vi "GEA3 HEWH Example.vi"() -> ()   [LabVIEW 2016]
uses:
  type defs/ERD Write Data In.ctl
  type defs/Data Type.ctl
  Type Definitions/GEA3 HEWH ERD Data.ctl
  Type Definitions/GEA3 HEWH Mixing Valve.ctl
  library/GEA2_Toolkit.lvlib
panel:
  in  "index":i32
  in  "Enable EMV List":bool
  out "ERD Data":string[][](array[string])
  out "Cycles":i32
  out "ERD Data":T1
  out "Raw Data Out":string
  in  "ERD Write Data In":T3 {"ERD Number" format="%.0x"}
  in  "Configure Send?":bool
  in  "stop":bool
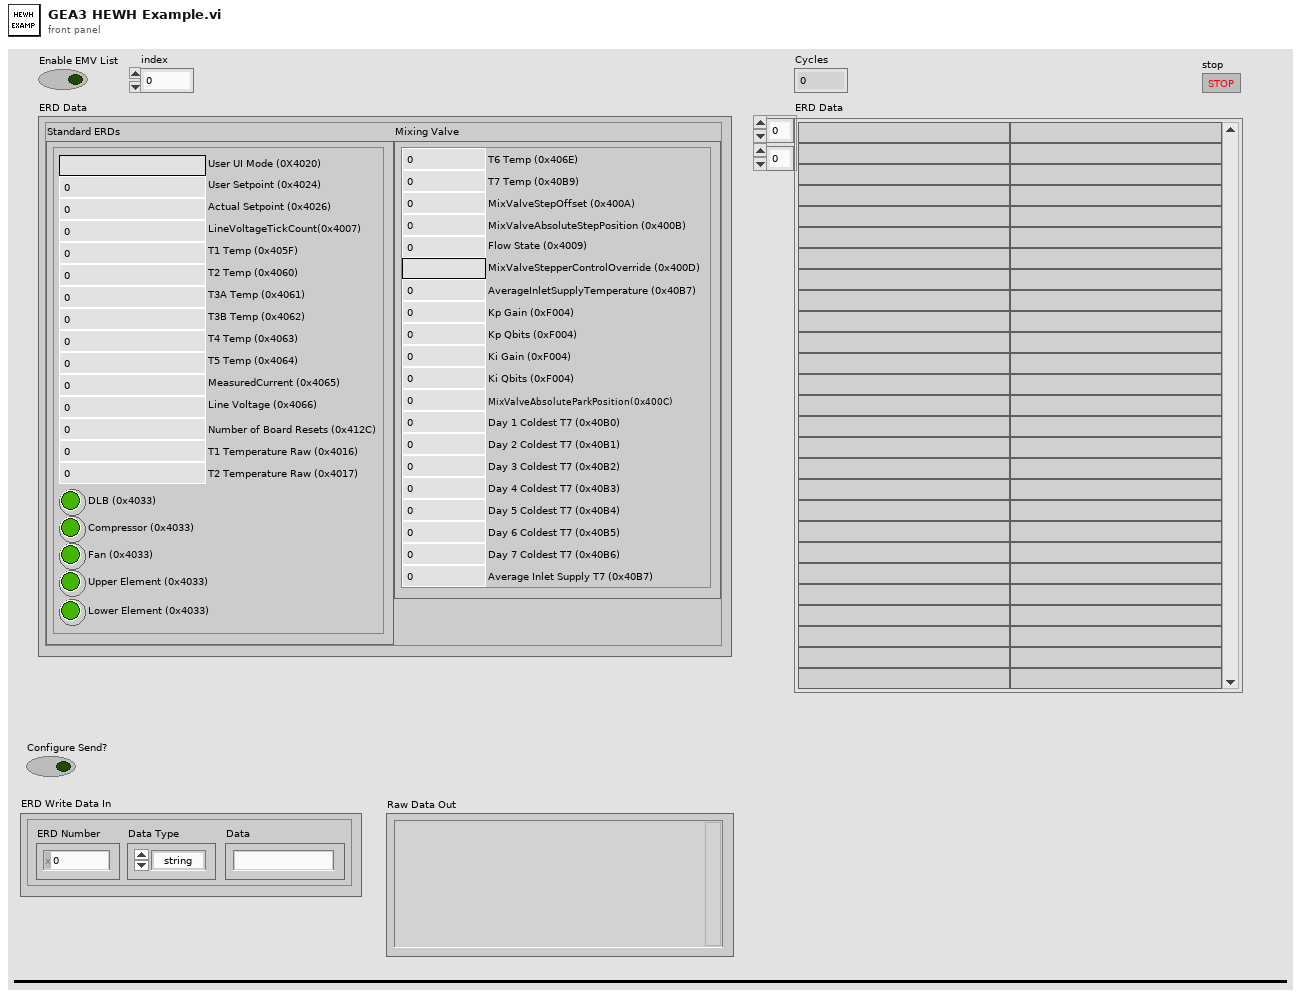
[diagram p1: front panel]
types:
  T1 = typedef "GEA3 HEWH ERD Data.ctl" = cluster{"Mixing Valve":T2, "Standard ERDs":cluster{"User UI Mode (0X4020)":string, "User Setpoint (0x4024)":u16, "Actual Setpoint (0x4026)":u16, "DLB (0x4033)":bool, "Compressor (0x4033)":bool, "Lower Element (0x4033)":bool, "Upper Element (0x4033)":bool, "Fan (0x4033)":bool, "T1 Temp (0x405F)":dbl, "T2 Temp (0x4060)":dbl, "T3A Temp (0x4061)":dbl, "T3B Temp (0x4062)":dbl, "T4 Temp (0x4063)":dbl, "T5 Temp (0x4064)":dbl, "Line Voltage (0x4066)":dbl, "MeasuredCurrent (0x4065)":dbl, "LineVoltageTickCount(0x4007)":u16, "Number of Board Resets (0x412C)":u16, "T1 Temperature Raw (0x4016)":u16, "T2 Temperature Raw (0x4017)":u16}}
  T2 = typedef "GEA3 HEWH Mixing Valve.ctl" = cluster{"T7 Temp (0x40B9)":dbl, "MixValveStepOffset (0x400A)":i16, "MixValveAbsoluteStepPosition (0x400B)":i16, "Flow State (0x4009)":u8, "MixValveStepperControlOverride (0x400D)":string, "AverageInletSupplyTemperature (0x40B7)":dbl, "T6 Temp (0x406E)":dbl, "Kp Gain (0xF004)":u16, "Kp Qbits (0xF004)":u16, "Ki Gain (0xF004)":u16, "Ki Qbits (0xF004)":u16, "MixValveAbsoluteParkPosition(0x400C)":i16, "Day 2 Coldest T7 (0x40B1)":dbl, "Day 1 Coldest T7 (0x40B0)":dbl, "Day 4 Coldest T7 (0x40B3)":dbl, "Day 3 Coldest T7 (0x40B2)":dbl, "Day 6 Coldest T7 (0x40B5)":dbl, "Day 5 Coldest T7 (0x40B4)":dbl, "Average Inlet Supply T7 (0x40B7)":dbl, "Day 7 Coldest T7 (0x40B6)":dbl}
  T3 = typedef "GEA2_Toolkit.lvlib/ERD Write Data In.ctl" = cluster{"ERD Number":u16, "Data Type":T4, "Data":string}
  T4 = typedef "GEA2_Toolkit.lvlib/Data Type.ctl" = enum16{"string", "boolean", "uint8_t", "uint16_t", "uint32_t", "uint64_t", "int8_t", "int16_t", "int32_t", "int64_t"}
  T5 = typedef "GEA2_Toolkit.lvlib/Source_Destination.ctl" = cluster{"Source":u8, "Destination":u8}
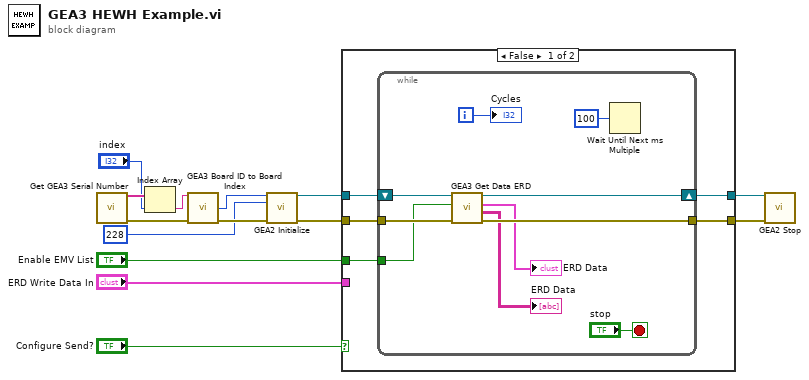
[diagram p0: block diagram]
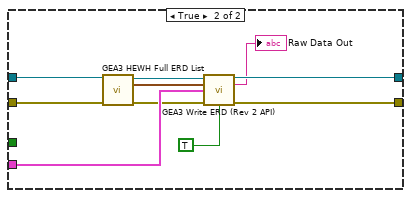
[diagram p2: hidden frame]
diagram:
  n1 = call "Get GEA3 Serial Number.vi"() -> ("GEA3 Serial Numbers"=w10:string[], "Error Out"=w11:errorcluster)  [unwired: 14 in]
  n2 = Index Array(array=w10, index="index") -> (element=w9:string)
  n3 = call "GEA3 Board ID to Board Index.vi"("GEA3 Serial Number"=w9, "Error In"=w11) -> ("Board Index"=w12:i32, "Error Out"=w13:errorcluster)  [unwired: 9 in, 3 out]
  n4 = call "GEA2 Initialize.vi"("Board Index"=w12, "Source Address"=u8 228, "error in"=w13) -> ("GEA2 Reference Out"=w5:refnum<k24>, "error out"=w1:errorcluster)  [unwired: 10 in, 1 out]
  n5 = case shown="False" "Configure Send?" {
    tunnel: w1 -> [w19 w34]
    tunnel: w5 -> [w18 w31]
    tunnel: [w17 w38] -> w14
    tunnel: [w16 w39] -> w8
    tunnel: "ERD Write Data In" -> [_ w35]
    tunnel: "Enable EMV List" -> [w15 _]
    frame False {
      n6 = while {
        shift-right: [w27] -> w17
        shift-left: w18 -> [w22]
        tunnel: w19 -> [w23]
        tunnel: [w26] -> w16
        tunnel: w15 -> [w20]
        i -> [w24]
        stop <- "stop" stop-if-true
        n7 = call "GEA3 Get Data ERD.vi"("error in (no error)"=w23, "Enable EMV List"=w20, ".NET Refnum in"=w22) -> ("error out"=w26:errorcluster, "ERD Data"=→"ERD Data":string[][], "ERD Data  2"=→"ERD Data":T1, ".NET Refnum out"=w27:refnum<k24>)  [unwired: 5 in]
        n8 = Wait Until Next ms Multiple(millisecond multiple=u32 100) -> ()  [unwired: 1 out]
        "Cycles" <- w24
      }
    }
    frame True {
      n9 = call "GEA3 HEWH Full ERD List.vi"("error in (no error)"=w34, "GEA2 Reference In"=w31) -> ("error out"=w33:errorcluster, "GEA Inputs"=w32:T5, "GEA2 Reference Out"=w30:refnum<k24>)  [unwired: 5 in, 2 out]
      n10 = call "GEA3 Write ERD (Rev 2 API).vi"("GEA2 Reference In"=w30, "GEA Inputs"=w32, "ERD Write Data In"=w35, "Error In"=w33, "Verify ERD Response?"=TRUE) -> ("GEA2 Reference Out"=w38:refnum<k24>, "Raw Data Out"=→"Raw Data Out":string, "Error Out"=w39:errorcluster)  [unwired: 7 in, 1 out]
    }
  }
  n11 = call "GEA2 Stop.vi"("GEA2 Reference In"=w14, "Error In"=w8) -> ()  [unwired: 13 in, 1 out]
